vi "EXCOM_SPAM.vi"() -> ()   [LabVIEW 2011]
panel:
  in  "Spam #22":bool
  in  "Spam #1":bool
  in  "Spam #28":bool
  in  "Spam #26":bool
  in  "Spam #25":bool
  out "Année":dbl format="%.2f"
  in  "TCS VRN IN 2":refnum<visa-resource-name>
  in  "Port Number 2":i32
  out "CommAct 2":bool
  in  "Equinox":dbl
  in  "Delay #2":u32
  in  "Delay #1":u32
  out "Error OUT":errorcluster
  out "CommAct":bool
  in  "stop":bool
  in  "Port Number":i32
  in  "TCS VRN IN":refnum<visa-resource-name>
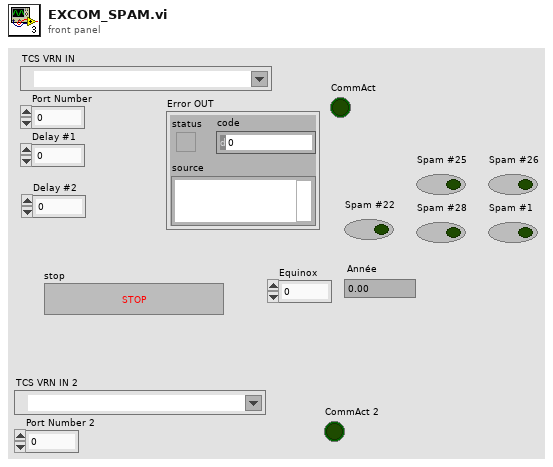
[diagram p1: front panel]
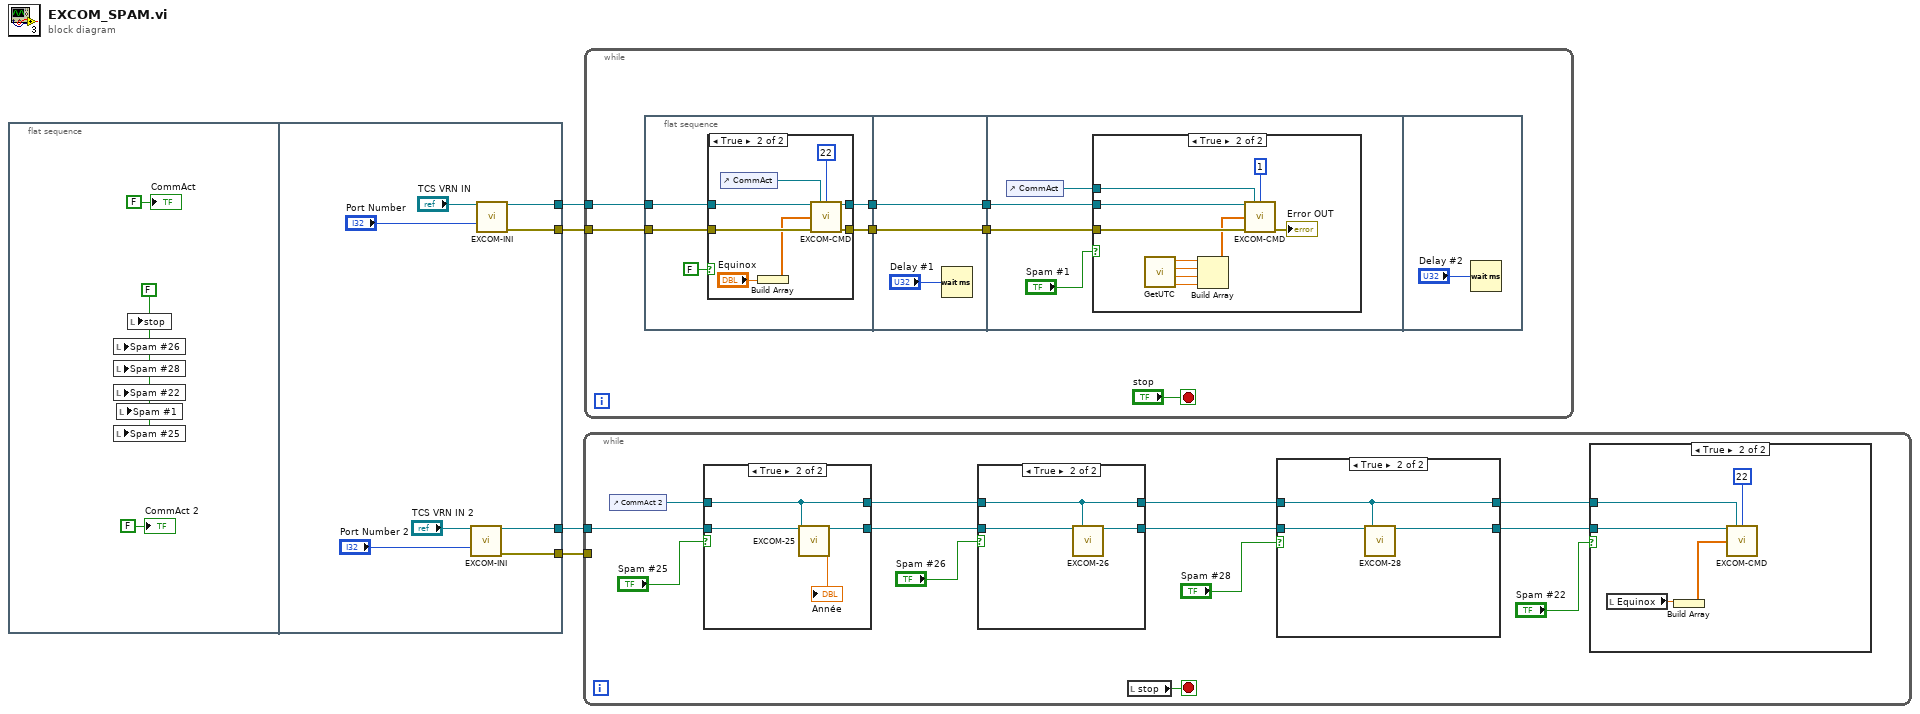
[diagram p0: block diagram]
diagram:
  n1 = flat-sequence {
    tunnel: [w15] -> w4
    tunnel: [w14] -> w3
    tunnel: [w13] -> w2
    tunnel: [w12] -> w1
    frame #0 {
      w7 = FALSE ("CommAct")
      n2 = local write "Spam #26"(w7) -> ()
      n3 = local write "Spam #28"(w7) -> ()
      n4 = local write "Spam #22"(w7) -> ()
      n5 = local write "Spam #25"(w7) -> ()
      n6 = local write "Spam #1"(w7) -> ()
      n7 = local write "stop"(w7) -> ()
      "CommAct 2" <- FALSE ("CommAct")
      "CommAct" <- FALSE ("CommAct")
    }
    frame #1 {
      n8 = call "EXCOM-INI.vi"("TCS VRN IN"="TCS VRN IN 2", "Port Number"="Port Number 2") -> ("TCS VRN OUT"=w13:refnum<visa-resource-name>, "error out"=w12:errorcluster)  [unwired: 12 in]
      n9 = call "EXCOM-INI.vi"("TCS VRN IN"="TCS VRN IN", "Port Number"="Port Number") -> ("TCS VRN OUT"=w15:refnum<visa-resource-name>, "error out"=w14:errorcluster)  [unwired: 12 in]
    }
  }
  n10 = while {
    tunnel: w2 -> [w27]
    tunnel: w1 -> [_]
    stop <- w28 stop-if-true
    n11 = control-ref of="CommAct 2"() -> (w25:refnum<vi>)
    n12 = case shown="True" "Spam #25" {
      tunnel: w27 -> [w44 w49]
      tunnel: w25 -> [w45 w47]
      tunnel: [w45 w47] -> w23
      tunnel: [w44 w46] -> w24
      frame False {
      }
      frame True {
        n13 = call "EXCOM-25.vi"("VISA resource name"=w49, "Bool Refnum"=w47) -> ("VISA resource name dup"=w46:refnum<visa-resource-name>, "Année"=→"Année":dbl)  [unwired: 3 in, 13 out]
      }
    }
    n14 = case shown="True" "Spam #26" {
      tunnel: w24 -> [w39 w43]
      tunnel: w23 -> [w40 w42]
      tunnel: [w40 w42] -> w21
      tunnel: [w39 w41] -> w20
      frame False {
      }
      frame True {
        n15 = call "EXCOM-26.vi"("VRN IN"=w43, "Bool Refnum"=w42) -> ("VRN OUT"=w41:refnum<visa-resource-name>)  [unwired: 7 in, 6 out]
      }
    }
    n16 = local read "stop"() -> (w28:bool)
    n17 = case shown="True" "Spam #28" {
      tunnel: w21 -> [w34 w36]
      tunnel: w20 -> [w35 w38]
      tunnel: [w35 w37] -> w17
      tunnel: [w34 w36] -> w16
      frame False {
      }
      frame True {
        n18 = call "EXCOM-28.vi"("VISA resource name"=w38, "Bool Refnum"=w36) -> ("VISA resource name dup"=w37:refnum<visa-resource-name>)  [unwired: 12 in, 5 out]
      }
    }
    n19 = case shown="True" "Spam #22" {
      tunnel: w17 -> [_ w31]
      tunnel: w16 -> [_ w29]
      frame False {
      }
      frame True {
        n20 = local read "Equinox"() -> (w30:dbl)
        n21 = Build Array(w30) -> (w33:dbl[])
        n22 = call "EXCOM-CMD.vi"("VRN IN"=w31, "Bool Refnum"=w29, "Commande #"=22, "Args"=w33) -> ()  [unwired: 9 in, 3 out]
      }
    }
  }
  n23 = while {
    tunnel: w4 -> [w56]
    tunnel: w3 -> [w55]
    stop <- "stop" stop-if-true
    n24 = flat-sequence {
      tunnel: w56 -> [w61]
      tunnel: w55 -> [w60]
      tunnel: [w59] -> w53
      tunnel: [w58] -> w52
      tunnel: w53 -> [w74]
      tunnel: w52 -> [w73]
      tunnel: [w74] -> w51
      tunnel: [w73] -> w50
      tunnel: w51 -> [w78]
      tunnel: w50 -> [w77]
      frame #0 {
        n25 = case shown="True" FALSE {
          tunnel: w61 -> [w62 w71]
          tunnel: w60 -> [w63 w70]
          tunnel: [w62 w68] -> w59
          tunnel: [w63 w67] -> w58
          frame False {
          }
          frame True {
            n26 = control-ref of="CommAct"() -> (w66:refnum<vi>)
            n27 = Build Array("Equinox") -> (w64:dbl[])
            n28 = call "EXCOM-CMD.vi"("VRN IN"=w71, "Bool Refnum"=w66, "Commande #"=22, "Args"=w64, "Error IN"=w70) -> ("VRN OUT"=w68:refnum<visa-resource-name>, "Error OUT"=w67:errorcluster)  [unwired: 8 in, 1 out]
          }
        }
      }
      frame #1 {
        n29 = Wait (ms)(milliseconds to wait="Delay #1") -> ()  [unwired: 1 out]
      }
      frame #2 {
        n30 = control-ref of="CommAct"() -> (w75:refnum<vi>)
        n31 = case shown="True" "Spam #1" {
          tunnel: w78 -> [_ w88]
          tunnel: w77 -> [_ w87]
          tunnel: w75 -> [_ w86]
          frame False {
          }
          frame True {
            n32 = call "GetUTC.vi"() -> ("UTC_fractional"=w80:dbl, "Day"=w81:dbl, "Month"=w82:dbl, "Year"=w83:dbl)  [unwired: 5 out]
            n33 = Build Array(w83, w82, w81, w80) -> (w79:dbl[])
            n34 = call "EXCOM-CMD.vi"("VRN IN"=w88, "Bool Refnum"=w86, "Commande #"=1, "Args"=w79, "Error IN"=w87) -> ("Error OUT"=→"Error OUT":errorcluster)  [unwired: 8 in, 2 out]
          }
        }
      }
      frame #3 {
        n35 = Wait (ms)(milliseconds to wait="Delay #2") -> ()  [unwired: 1 out]
      }
    }
  }
